vi "_ServerDemo.vi"() -> ()   [LabVIEW 2010]
uses:
  <vilib>/Utility/cursorutil.llb/Set Cursor (Icon Pict).vi
panel:
  out "ScanCode":i16
  out "selection":i32=-1
  out "Boundaries":cluster{i32, i32}[](array[cluster])=[{10, 22}, {30, 42}, {50, 62}]
  in  "Done":bool
  in  "Symbols":T1(array[ring])
  in  "Server Names":string[](array[string])
  out "2D Picture":picture
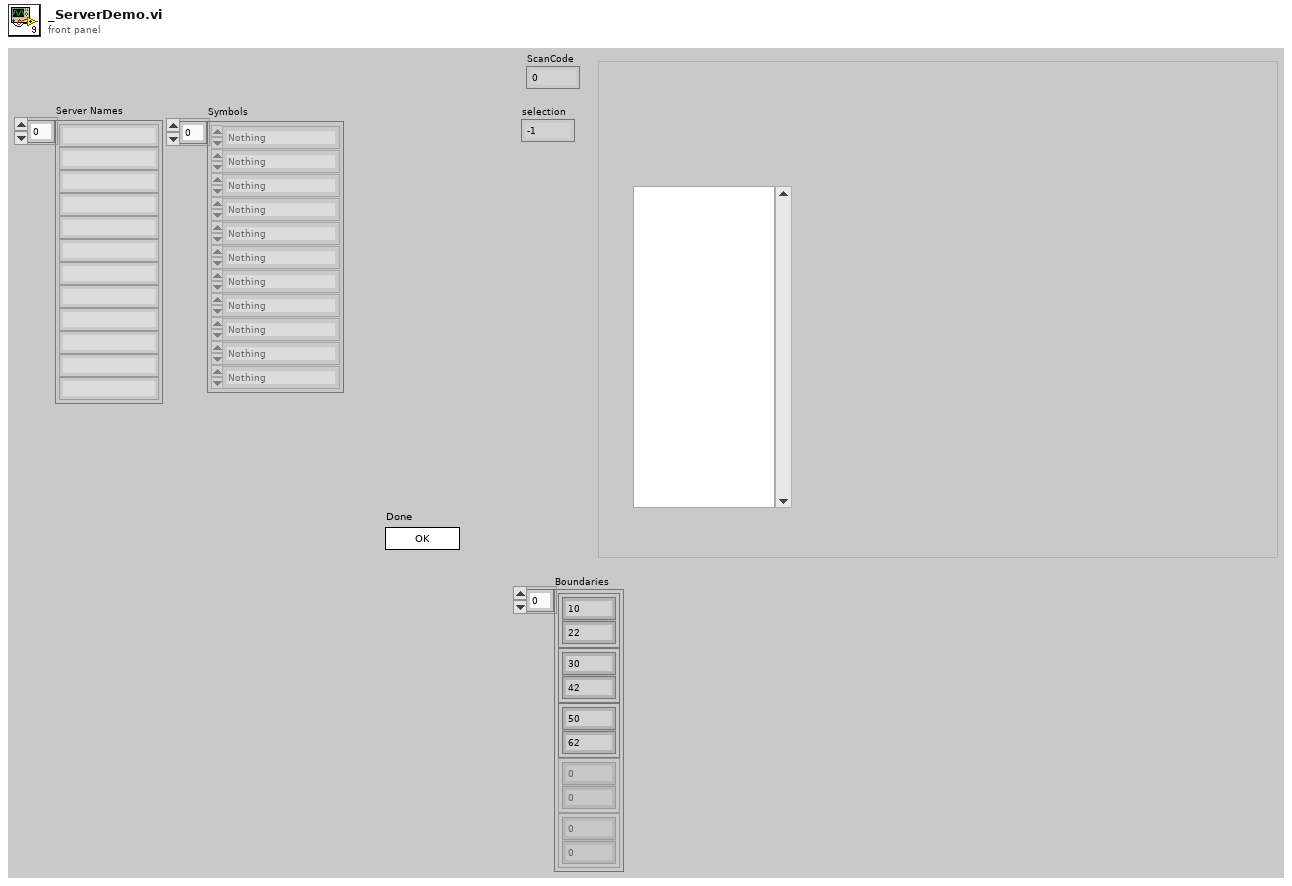
[diagram p1: front panel]
types:
  T1 = enum16{"Nothing", "Not Connected", "Registered", "Connected"}[]
  T2 = typedef "LVMouseTypeDef.ctl" = cluster{"Mouse Position":cluster{"X":i32, "Y":i32}, "Mouse Modifiers":cluster{"Button Down":bool, "Shift Mod":bool, "Menu Mod":bool, "Option Mod":bool}}
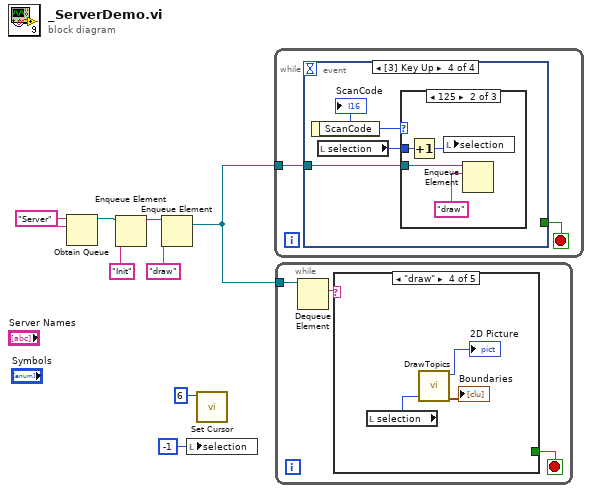
[diagram p0: block diagram]
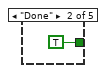
[diagram p3: hidden frame]
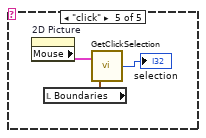
[diagram p5: hidden frame]
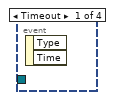
[diagram p6: hidden frame]
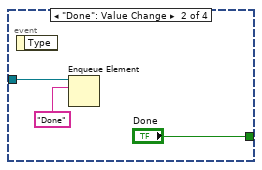
[diagram p7: hidden frame]
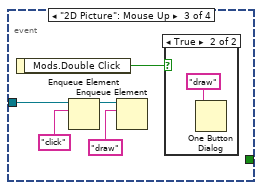
[diagram p8: hidden frame]
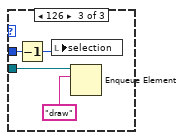
[diagram p11: hidden frame]
diagram:
  w7 = "Server" ("name (unnamed)")
  n1 = Obtain Queue(name (unnamed)=w7, element data type=w7) -> (queue out=w8:refnum<queue>)  [unwired: 3 in, 2 out]
  n2 = Enqueue Element(queue=w8, element="Init") -> (queue out=w5:refnum<queue>)  [unwired: 2 in, 2 out]
  n3 = Enqueue Element(queue=w5, element="draw") -> (queue out=w4:refnum<queue>)  [unwired: 2 in, 2 out]
  n4 = local write "selection"(-1 ("selection")) -> ()
  n5 = call-poly <vilib>:"Set Cursor.vi"("icon"=u16 6) -> ()  [unwired: 9 in, 2 out]
  n6 = while {
    tunnel: w4 -> [w9]
    stop <- w10 stop-if-true
    n7 = event shown="[3] Key Up" {
      selector: _ -> [_ _ _ _]
      dyn-events: _ -> [_ _ _ _]
      timeout: _ -> [_ _ _ _]
      tunnel: [_ "Done" _ _] -> w10
      tunnel: w9 -> [_ w12 w18 w22]
      event Timeout {
        n8 = event-data() -> ()  [unwired: 1 in, 2 out]
      }
      event "Done": Value Change {
        n9 = event-data() -> ()  [unwired: 1 in, 1 out]
        n10 = Enqueue Element(queue=w12, element="Done" ("name (unnamed)")) -> ()  [unwired: 2 in, 3 out]
      }
      event "2D Picture": Mouse Up {
        n11 = event-data() -> ("Mods.Double Click"=w14:bool)  [unwired: 1 in]
        n12 = Enqueue Element(queue=w18, element="click" ("name (unnamed)")) -> (queue out=w16:refnum<queue>)  [unwired: 2 in, 2 out]
        n13 = Enqueue Element(queue=w16, element="draw" ("name (unnamed)")) -> ()  [unwired: 2 in, 3 out]
        n14 = case shown="True" w14 {
          frame False {
          }
          frame True {
            n15 = One Button Dialog(message="draw" ("name (unnamed)")) -> ()  [unwired: 1 in, 1 out]
          }
        }
      }
      event Key Up {
        n16 = event-data() -> ("ScanCode"=w21:i16)  [unwired: 1 in]
        "ScanCode" <- w21
        n17 = local read "selection"() -> (w20:i32)
        n18 = case shown="125" w21 {
          tunnel: w22 -> [_ w23 w27]
          tunnel: w20 -> [_ w25 w29]
          frame 0, Default {
          }
          frame 125 {
            n19 = Increment(x=w25) -> (x+1=w24:i32)
            n20 = local write "selection"(w24) -> ()
            n21 = Enqueue Element(queue=w23, element="draw" ("name (unnamed)")) -> ()  [unwired: 2 in, 3 out]
          }
          frame 126 {
            n22 = Decrement(x=w29) -> (x-1=w28:i32)
            n23 = local write "selection"(w28) -> ()
            n24 = Enqueue Element(queue=w27, element="draw" ("name (unnamed)")) -> ()  [unwired: 2 in, 3 out]
          }
        }
      }
    }
  }
  n25 = while {
    tunnel: w4 -> [w33]
    stop <- w31 stop-if-true
    n26 = Dequeue Element(queue=w33) -> (element=w32:string)  [unwired: 2 in, 3 out]
    n27 = case shown="\"draw\"" w32 {
      tunnel: [_ TRUE _ _ _] -> w31
      frame "False", Default {
      }
      frame "Done" {
      }
      frame "Init" {
      }
      frame "draw" {
        n28 = local read "selection"() -> (w35:i32)
        n29 = call "DrawTopics.vi"("Selection"=w35) -> ("new picture"=→"2D Picture":picture, "Boundaries"=→"Boundaries":cluster{i32, i32}[])  [unwired: 2 in, 2 out]
      }
      frame "click" {
        n30 = property on="2D Picture" class="Pict"() -> ("Mouse"=w39:T2)  [unwired: 2 in, 2 out]
        n31 = local read "Boundaries"() -> (w38:cluster{i32, i32}[])
        n32 = call "GetClickSelection.vi"("Boundaries"=w38, "Mouse"=w39) -> ("selection"=→"selection":i32)
      }
    }
  }
